vi "Tmp_M submodule.vi"() -> (0 "Error Out":errorcluster, 3 "Temperatures":T2[](array[typedef]) {"Time stamp" format="%<%H:%M:%S%2u\n%Y/%m/%d>T"})   [LabVIEW 2021, in "Temperature monitor.lvlib"]
doc: "Magnet module controls: power supply unit (PSU/SMS) and temperature monitor (TM/LSC218).\nPSU controls mainly: switch heater and ramping of current which runs throught coil.\nTM controls temperature of switch, coil and cryostat.\nMessage for magnet is a cluster that contains: {(enum) Command , (variant) Data}\nFor simplifieing of documentation, the Command is noted as a name of instruction, and Data is represented by a requered datatype (mostly cluster) name.\nCommands:\nInitialize(Magnet Config Constants) - Sugesstion: Load configuration constants from configuration file.\nSet field (Set field{B, R, cr}) - B-field[T], R-ramp[A/s], cr - custom ramp[bool].\nSwitch mode(mode) - to persistant, or to ramping.\nBlackout() - undone functionality of emergency deenergizing.\nUpdate() - Important! This triggers update of data from instruments. Shoud occure in regular intervals as priority message.\nResponses:\nMagnet initialized ();\nTM revision(temperature monitor revision);\nMagnet init error(error);\nSetting field(Set Field{B, R, cr});\nWarning(string);\nSwitching to(mode);\nUpdate error(error);\nTM update(TM sensors);\nPSU update(PSU data);\nMagnet status();"
uses:
  Temperature monitor.lvlib
  ctl/Cryostat temperature sensors.ctl
  Magnet module.lvlib
  Messenger service/Data types/Module name.ctl
  Messenger service/MessengerLib.lvlib
  ctl/TM states.ctl
  <userlib>/MatS libs/MatS Messenger/Queued messenger.lvlib
  <userlib>/MatS libs/MatS Messenger/TypeDefs/Mailbox ref.ctl
  Typedefs/TM_status.ctl
  <userlib>/MatS libs/MatS Messenger/TypeDefs/General message.ctl
  Typedefs/Tmp_M commands.ctl
panel:
  in  "timeout ms":i32
  in  "Instr VISA ref":refnum<visa-resource-name>
  in  "This module":T1
  in  "Supra module":T1
  out "Connected":bool
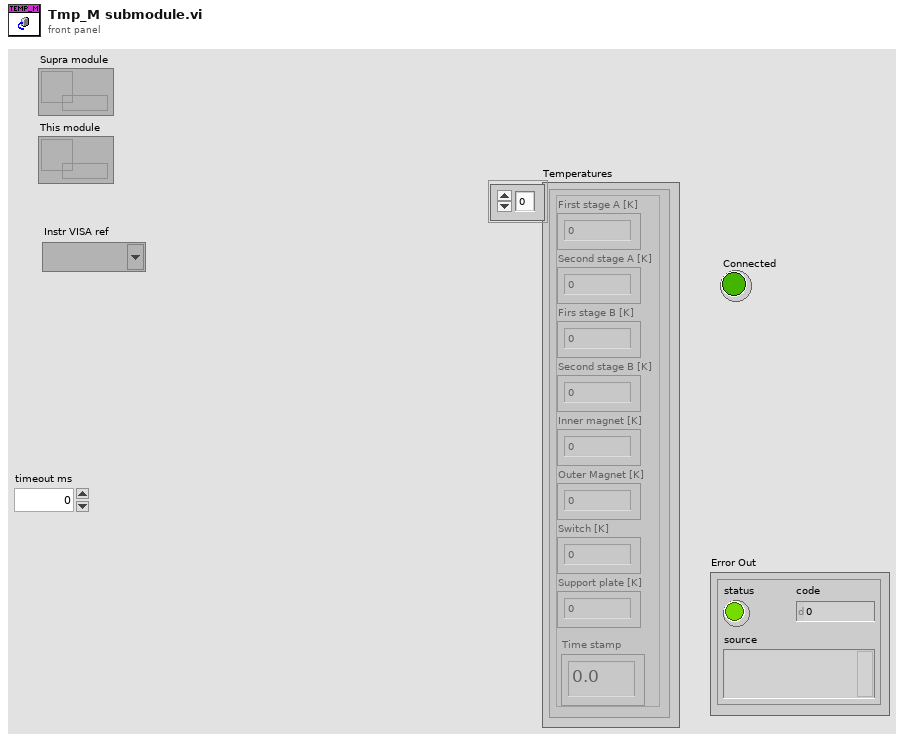
[diagram p1: front panel]
types:
  T1 = typedef "Queued messenger.lvlib/Mailbox ref.ctl" = refnum<queue>
  T2 = typedef "Magnet module.lvlib/Cryostat temperature sensors.ctl" = cluster{"First stage A [K]":dbl, "Second stage A [K]":dbl, "Firs stage B [K]":dbl, "Second stage B [K]":dbl, "Inner magnet [K]":dbl, "Outer Magnet [K]":dbl, "Switch [K]":dbl, "Support plate [K]":dbl, "Time stamp":dbl}
  T3 = typedef "Temperature monitor.lvlib/Tmp_M commands.ctl" = enum16{"Ignore", "Log", "Connect", "Set timeout", "Update", "Disconnect", "End"}
  T4 = typedef "Temperature monitor.lvlib/TM_status.ctl" = cluster{"Supramodule":T1, "This module":T1, "Module name":string, "Standalone?":bool, "Stopped?":bool, "Instr VISA ref":refnum<visa-resource-name>, "Connected?":bool, "Last update":timestamp, "Logs":string[]}
  T5 = typedef "TM states.ctl" = enum16{"Initialize", "Wait for event", "Check message", "End"}
  T6 = typedef "Queued messenger.lvlib/General message.ctl" = cluster{"Sender":string, "Recipient":string, "Topic":string, "Content":variant, "Time Stamp":timestamp}
  T7 = typedef "MessengerLib.lvlib/Module name.ctl" = enum16{"Emty", "Magnet", "VTI", "Excitation", "Servo", "Acquisition", "Rotator", "Digitizer", "SMU2450", "Carousel", "Multimeter", "Tmp monitor", "Power monitor"}
  T8 = enum32{"Bad", "Idle", "Run top level", "Running"}
  T9 = typedef "MessengerLib.lvlib/Mailbox address.ctl" = refnum<queue>
  T10 = typedef "Temperature monitor.lvlib/TM Revision.ctl" = cluster{"Instr Serial Number":string, "Instr Driver Revision":string, "Instr Firmware Revision":string, "Instr Model Number":string}
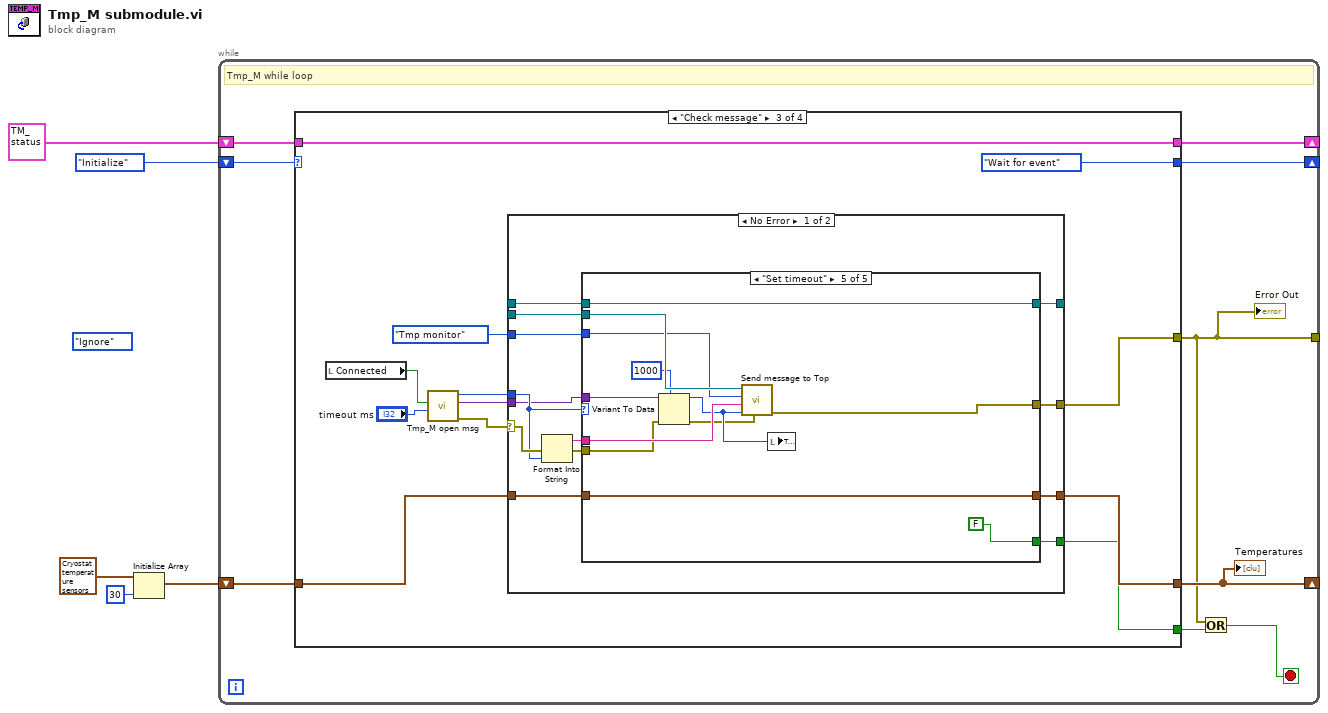
[diagram p0: block diagram]
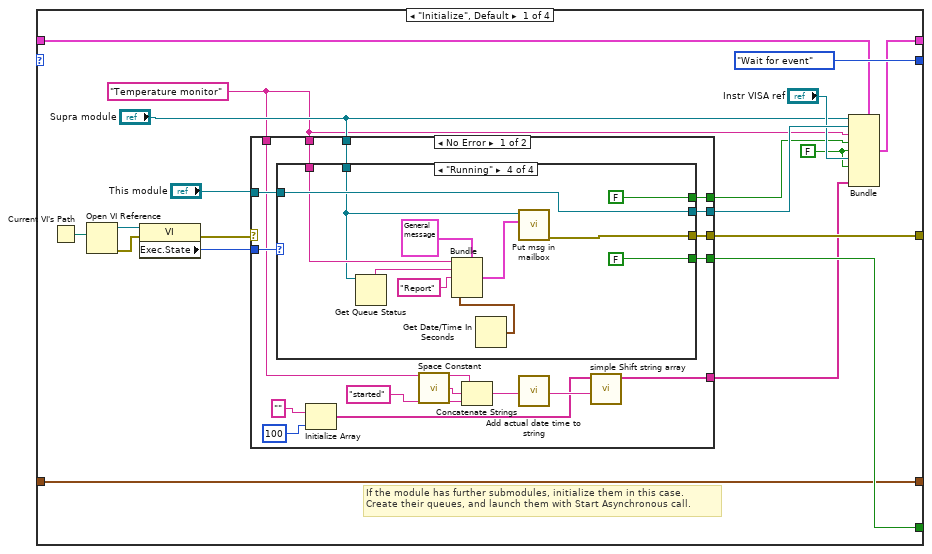
[diagram p2: hidden frame]
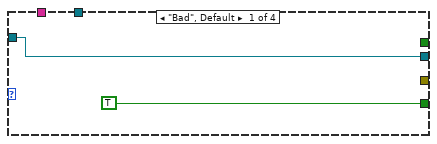
[diagram p3: hidden frame]
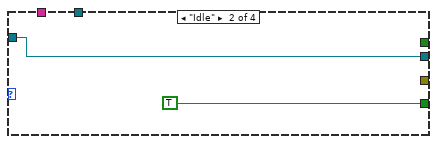
[diagram p4: hidden frame]
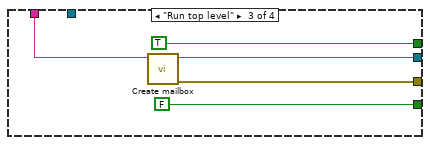
[diagram p5: hidden frame]
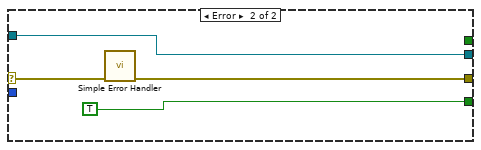
[diagram p6: hidden frame]
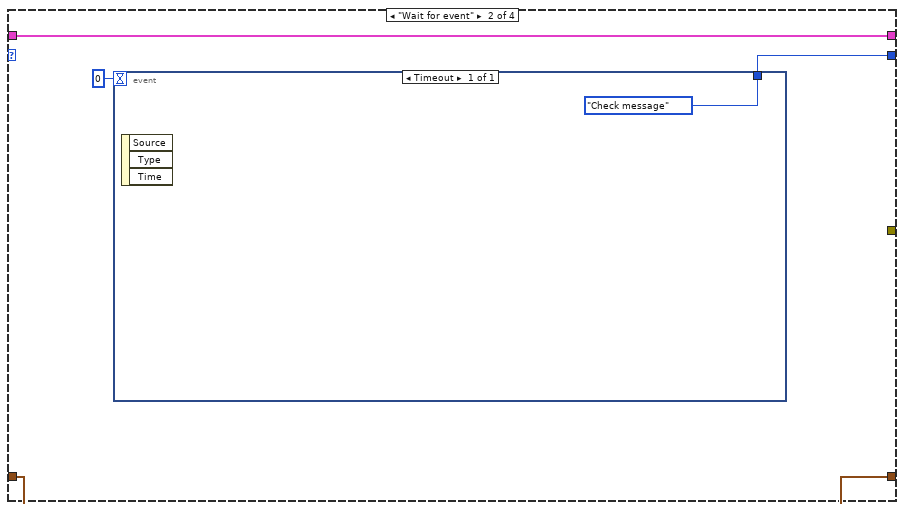
[diagram p7: hidden frame]
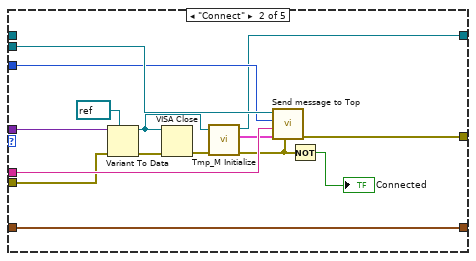
[diagram p9: hidden frame]
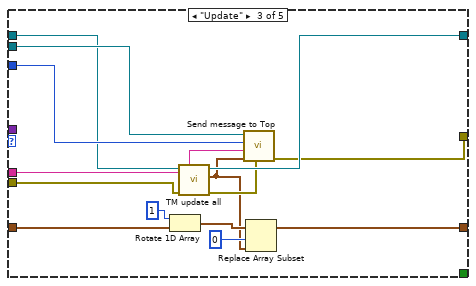
[diagram p10: hidden frame]
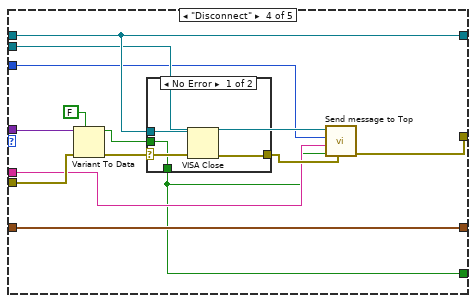
[diagram p11: hidden frame]
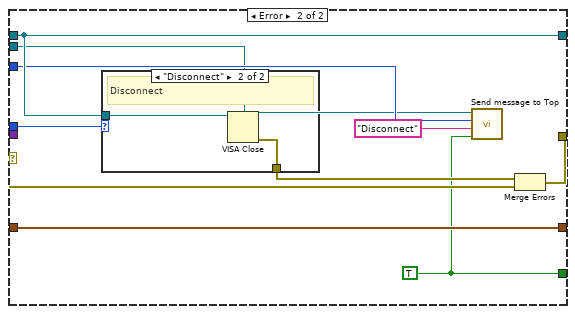
[diagram p13: hidden frame]
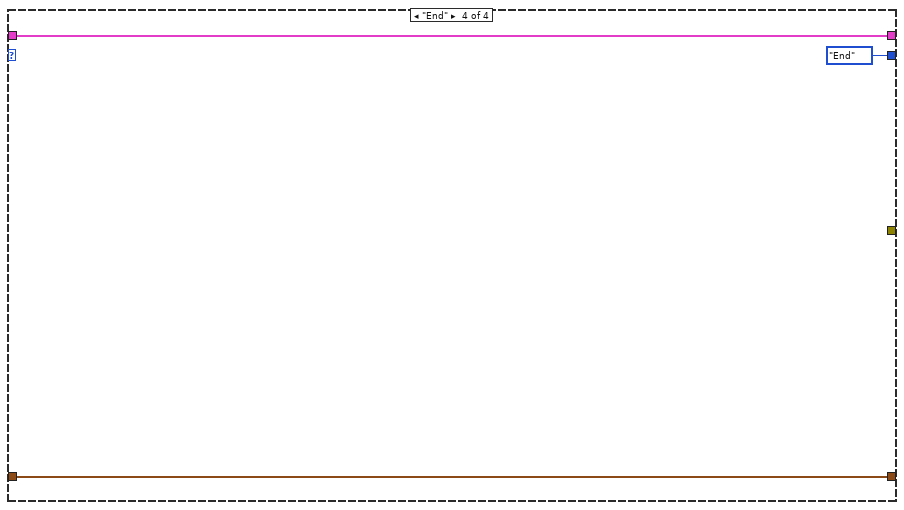
[diagram p15: hidden frame]
diagram:
  (unwired) Tmp_M_commands."Ignore" ("Command")
  n1 = Initialize Array(T2 {"First stage A [K]"=0.0, "Second stage A [K]"=0.0, "Firs stage B [K]"=0.0, "Second stage B [K]"=0.0, "Inner magnet [K]"=0.0, "Outer Magnet [K]"=0.0, "Switch [K]"=0.0, "Support plate [K]"=0.0, "Time stamp"=0.0} ("LSC218 sensors"), 30 ("dimension size")) -> (w5:T2[])
  n2 = while {
    shift-right: [w13] -> _
    shift-left: w5 -> [w14]
    tunnel: [w7] -> _
    shift-right: [w10] -> _
    shift-left: TM_states."Initialize" -> [w11]
    shift-right: [w6] -> _
    shift-left: T4 {"Supramodule"=refnum, "This module"=refnum, "Module name"="", "Standalone?"=FALSE, "Stopped?"=FALSE, "Instr VISA ref"="", "Connected?"=FALSE, "Last update"=timestamp(0 s since 1904-01-01), "Logs"=[]} ("Temperature monitor status") -> [w9]
    stop <- w8 stop-if-true
    # "Tmp_M while loop"
    n3 = case shown="\"Check message\"" w11 {
      tunnel: w14 -> [w23 w75 w94 w183]
      tunnel: [w23 w75 w93 w183] -> w13
      tunnel: [w28 _ w86 _] -> w12
      tunnel: [w26 _ w83 _] -> w7
      tunnel: [TM_states."Wait for event" w78 TM_states."Wait for event" TM_states."End"] -> w10
      tunnel: w9 -> [w27 w76 w81 w184]
      tunnel: [w24 w76 w81 w184] -> w6
      frame "Initialize", Default {
        w17 = "Temperature monitor" ("name (unnamed)")
        w20 = FALSE ("Connected?")
        # "If the module has further submodules, initialize them in this case.\nCreate their queues, and launch them with Start Asynchronous call."
        n4 = Current VI's Path() -> (path=w31:path)
        n5 = Open VI Reference(vi path=w31) -> (vi reference=w32:refnum<vi>, error out=w30:errorcluster)  [unwired: 5 in]
        n6 = property class="VI"(reference=w32, error in=w30) -> (error out=w15:errorcluster, "Exec.State"=w29:T8)  [unwired: 1 out]
        n7 = case shown="No Error" w15 {
          selector: w15 -> [_ w73]
          tunnel: w29 -> [w50 _]
          tunnel: [w49 TRUE] -> w28
          tunnel: [w48 w72] -> w25
          tunnel: "This module" -> [w47 w72]
          tunnel: [w46 _] -> w21
          tunnel: [w45 w71] -> w26
          tunnel: w17 -> [w44 _]
          tunnel: "Supra module" -> [w43 _]
          tunnel: w17 -> [w39 _]
          tunnel: [w37 _] -> w16
          frame No Error {
            n8 = case shown="\"Running\"" w50 {
              tunnel: [TRUE TRUE FALSE FALSE] -> w49
              tunnel: [w51 w53 w58 w69] -> w48
              tunnel: w47 -> [w51 w53 _ w69]
              tunnel: [_ _ TRUE FALSE] -> w46
              tunnel: [_ _ w56 w63] -> w45
              tunnel: w44 -> [_ _ w55 w64]
              tunnel: w43 -> [_ _ _ w62]
              frame "Bad", Default {
              }
              frame "Idle" {
              }
              frame "Run top level" {
                n9 = call <userlib>:"Create mailbox.vi"("name (unnamed)"=w55) -> ("error out"=w56:errorcluster, "Mailbox ref"=w58:T1)  [unwired: 4 in, 1 out]
              }
              frame "Running" {
                n10 = Get Queue Status(queue=w62) -> (queue name=w61:string)  [unwired: 2 in, 7 out]
                n11 = Get Date/Time In Seconds() -> (seconds since 1Jan1904=w65:timestamp)
                n12 = Bundle(cluster=T6 {"Sender"="", "Recipient"="", "Topic"="", "Content"=variant, "Time Stamp"=timestamp(0 s since 1904-01-01)} ("Message"), "Sender"=w64, "Recipient"=w61, "Topic"="Report", "Time Stamp"=w65) -> (w66:T6)  [unwired: 1 in]
                n13 = call <userlib>:"Put msg in mailbox.vi"("Message"=w66, "Mailbox ref in"=w62) -> ("error out"=w63:errorcluster)  [unwired: 7 in, 2 out]
              }
            }
            n14 = Initialize Array("", 100 ("dimension size")) -> (w34:string[])
            n15 = call <vilib>:"Space Constant.vi"() -> ("String"=w42:string)
            n16 = Concatenate Strings(w39, w42, "started") -> (w40:string)
            n17 = call <userlib>:"Add actual date time to string.vi"("String in"=w40) -> ("String out"=w41:string)  [unwired: 4 in]
            n18 = call <userlib>:"simple Shift string array.vi"("Element in"=w41, "Array in"=w34) -> ("Array out"=w37:string[])  [unwired: 8 in, 1 out]
          }
          frame Error {
            n19 = call <vilib>:"Simple Error Handler.vi"("error in (no error)"=w73) -> ("error out"=w71:errorcluster)  [unwired: 4 in, 4 out]
          }
        }
        n20 = Bundle(cluster=w27, "Supramodule"="Supra module", "This module"=w25, "Module name"=w17, "Standalone?"=w21, "Stopped?"=w20, "Instr VISA ref"="Instr VISA ref", "Connected?"=w20, "Logs"=w16) -> (w24:T4)  [unwired: 1 in]
      }
      frame "Wait for event" {
        n21 = event shown="[0] Timeout" {
          selector: _ -> [_]
          dyn-events: _ -> [_]
          timeout: 0 -> [_]
          tunnel: [TM_states."Check message"] -> w78
          event Timeout {
            n22 = event-data() -> ()  [unwired: 1 in, 3 out]
          }
        }
      }
      frame "Check message" {
        n23 = local read "Connected"() -> (w84:bool)
        n24 = call "Tmp_M open msg.vi"("timeout ms (1000)"="timeout ms", "Connected"=w84) -> ("error out"=w88:errorcluster, "Data"=w87:variant, "Command"=w89:T3, "Queue in"=w90:T9)  [unwired: 4 in, 2 out]
        n25 = case shown="No Error" w88 {
          selector: w88 -> [w101 w175]
          tunnel: [w108 w173] -> w95
          tunnel: w89 -> [w100 w179]
          tunnel: w94 -> [w107 w180]
          tunnel: [w106 w180] -> w93
          tunnel: [w97 w171] -> w86
          tunnel: [w104 w178] -> w92
          tunnel: [w103 w178] -> w91
          tunnel: w87 -> [w99 _]
          tunnel: [w98 w177] -> w83
          tunnel: Module_name."Tmp monitor" ("Module") -> [w96 w174]
          frame No Error {
            n26 = Format Into String(error in=w101, w100) -> (resulting string=w105:string, error out=w102:errorcluster)  [unwired: 2 in]
            n27 = case shown="\"Set timeout\"" w100 {
              tunnel: w108 -> [_ w126 w136 w145 w169]
              tunnel: w107 -> [w111 w125 w140 w153 w170]
              tunnel: [w111 w125 w139 w153 w170] -> w106
              tunnel: w96 -> [_ w122 w137 w144 w166]
              tunnel: w105 -> [_ w123 w138 w143 w167]
              tunnel: [_ _ _ w141 FALSE] -> w97
              tunnel: [w110 w119 w134 w152 w165] -> w104
              tunnel: w103 -> [w110 _ w135 w152 w165]
              tunnel: w102 -> [w109 w115 w127 w149 w162]
              tunnel: w99 -> [_ w114 _ w150 w163]
              tunnel: [w109 w113 w133 w146 w159] -> w98
              frame "Ignore", Default {
              }
              frame "Connect" {
                n28 = Variant To Data(error in=w115, type=refnum<visa-resource-name> refnum ("LSC218"), Variant=w114) -> (data=w118:refnum<visa-resource-name>, error out=w124:errorcluster)
                n29 = VISA Close(VISA resource name=w118, error in (no error)=w124) -> (error out=w121:errorcluster)
                n30 = call "Tmp_M Initialize.vi"("error in (no error)"=w121, "VISA Refnum in"=w118) -> ("error out"=w116:errorcluster, "TM Revision"=w120:T10, "VISA Refnum out"=w119:refnum<visa-resource-name>)  [unwired: 7 in]
                n31 = call "Send message to Top.vi"("Error in (no error)"=w116, "Data"=w120, "Response"=w123, "Module"=w122, "Mailbox address in"=w126) -> ("Error out"=w113:errorcluster)  [unwired: 5 in, 1 out]
                n32 = Not(x=w116) -> (.not. x?=→"Connected":bool)
              }
              frame "Update" {
                n33 = Rotate 1D Array(1:w140, 2:1 ("n")) -> (0:w131:T2[])
                n34 = call "TM update all.vi"("error in (no error)"=w127, "VISA Refnum in"=w135) -> ("error out"=w129:errorcluster, "LSC218 sensors"=w128:T2, "VISA Refnum out"=w134:refnum<visa-resource-name>)  [unwired: 7 in]
                n35 = call "Send message to Top.vi"("Error in (no error)"=w129, "Data"=w128, "Response"=w138, "Module"=w137, "Mailbox address in"=w136) -> ("Error out"=w133:errorcluster)  [unwired: 5 in, 1 out]
                n36 = Replace Array Subset(array=w131, new element=w128, index=0) -> (w139:T2[])
              }
              frame "Disconnect" {
                n37 = Variant To Data(error in=w149, type=FALSE, Variant=w150) -> (data=w142:bool, error out=w148:errorcluster)
                n38 = case shown="No Error" w148 {
                  selector: w148 -> [w156 w158]
                  tunnel: w152 -> [w157 _]
                  tunnel: [w155 w158] -> w147
                  tunnel: w142 -> [w154 _]
                  tunnel: [w154 _] -> w141
                  frame No Error {
                    n39 = VISA Close(VISA resource name=w157, error in (no error)=w156) -> (error out=w155:errorcluster)
                  }
                  frame Error {
                  }
                }
                n40 = call "Send message to Top.vi"("Error in (no error)"=w147, "Data"=w141, "Response"=w143, "Module"=w144, "Mailbox address in"=w145) -> ("Error out"=w146:errorcluster)  [unwired: 5 in, 1 out]
              }
              frame "Set timeout" {
                n41 = Variant To Data(error in=w162, type=1000 ("timeout ms"), Variant=w163) -> (data=w161:i32, error out=w160:errorcluster)
                n42 = call "Send message to Top.vi"("Error in (no error)"=w160, "Data"=w161, "Response"=w167, "Module"=w166, "Mailbox address in"=w169) -> ("Error out"=w159:errorcluster)  [unwired: 5 in, 1 out]
                n43 = local write item#-1(w161) -> ()
              }
            }
          }
          frame Error {
            w171 = TRUE
            n44 = case shown="\"Disconnect\"" w179 {
              tunnel: w178 -> [_ w182]
              tunnel: [_ w181] -> w176
              frame "Ignore", Default {
                # "Nohing"
              }
              frame "Disconnect" {
                # "Disconnect"
                n45 = VISA Close(VISA resource name=w182) -> (error out=w181:errorcluster)  [unwired: 1 in]
              }
            }
            n46 = call "Send message to Top.vi"("Data"=w171, "Response"="Disconnect", "Module"=w174, "Mailbox address in"=w173) -> ()  [unwired: 6 in, 2 out]
            n47 = Merge Errors(w176, w175) -> (w177:errorcluster)
          }
        }
      }
      frame "End" {
      }
    }
    "Temperatures" <- w13
    "Error Out" <- w7
    n48 = Or(x=w7, y=w12) -> (x .or. y?=w8:bool)
  }
